vi "SS2 Live_Settings Storage.vi"(6 "Set/Get(F)":bool, 8 "Error In":errorcluster, 10 "Variant Data in":variant, 11 "Settings List":T8) -> (0 "Error Out":errorcluster, 2 "Variant Data out":variant)   [LabVIEW 2019]
uses:
  SS2 Live_Settings List.ctl
  SS2 DAQ Parameters 2.ctl
  SS2 Gate Definition.ctl
  SS2 Live_File Information.ctl
  SS2 Gate Configuration.ctl
  SS2 Live_Image ROI Information.ctl
  Phasor/Image Binning Options.ctl
  281105eb-bd69-41f7-a288-d5f8cce70846.vi
panel:
  in  "Tab Control":T1(tab)
  in  "Bitfile Version":string
  in  "BitFile Path":path
  in  "Buffer Size (# Gates)":u32=1 min=1
  in  "SS2 DAQ Parameters":T2 {"Laser Period" min=0.0 max=4.294967295}
  in  "Gate Configuration Definitions":T4[](array[typedef])
  in  "Image Binning Options":T5={"Use Image Binning"=FALSE, "X Bin"=1, "Y Bin"=1} {"Y Bin" min=1; "X Bin" min=1}
  in  "Image ROI Information":T6
  in  "# Datasets in Series":i32=1 min=1
  in  "File Information":T7
  in  "# Histogram Bins":i32=1 min=1 step=1
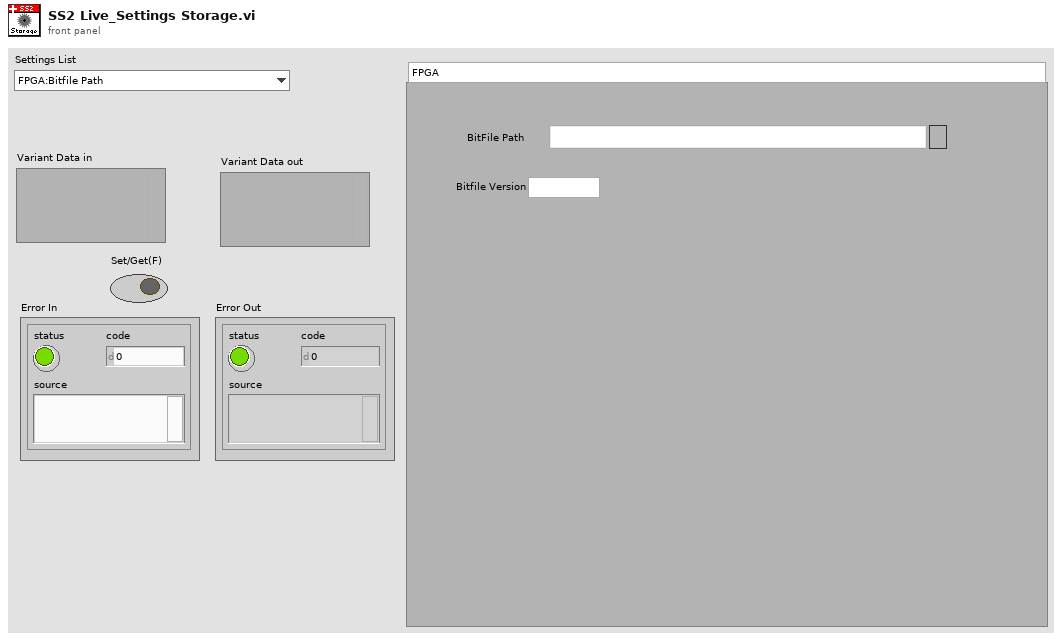
[diagram p1: front panel]
types:
  T1 = enum32{"FPGA", "Acquisition Parameters", "Image Parameters", "File Information", "UI Parameters"}
  T2 = typedef "SS2 DAQ Parameters 2.ctl" = cluster{"10 bits":bool, "# Exposure Sequences":u32, "# 1-bit Frame per Gate":u32, "Gate Shift":u32, "# Gates per Set":u32, "# Sets":u32, "Laser Period":dbl[unit], "Gate Offset":u32, "Auto-adjust Gate Offset":bool, "Gate Definition":T3}
  T3 = typedef "SS2 Gate Definition.ctl" = cluster{"gs_psincdec_0":u32, "gs_psincdec_1":u32, "gs_psincdec_2":u32, "gs_psincdec_3":u32, "gs_no_shift_adj_1":u32, "gs_no_shift_adj_2":u32, "gs_no_shift_adj_3":u32}
  T4 = typedef "SS2 Gate Configuration.ctl" = cluster{"Gate Configuration":string, "Gate Offset":u32, "Gate Definition":T3}
  T5 = typedef "Image Binning Options.ctl" = cluster{"Use Image Binning":bool, "X Bin":i32, "Y Bin":i32}
  T6 = typedef "SS2 Live_Image ROI Information.ctl" = cluster{"Save ROI Only":bool, "Left":u16, "Top":u16, "Right":u16, "Bottom":u16, "Use Current ROI":bool}
  T7 = typedef "SS2 Live_File Information.ctl" = cluster{"File Folder":path, "File Name":string, "File Index":u32, "Author":string, "Sample":string, "Compression":bool}
  T8 = typedef "SS2 Live_Settings List.ctl" = enum16{"FPGA:Bitfile Path", "FPGA:Bitfile Version", "Acquisition Parameters:SS2 DAQ Parameters", "Acquisition Parameters:Gate Configuration Array", "Acquisition Parameters:Buffer Size (# Gates)", "File Information:File Information", "File Information:# Datasets in Series", "Image Parameters:Image ROI Information", "Image Parameters:Image Binning Options", "UI Parameters:Histogram Bins Number"}
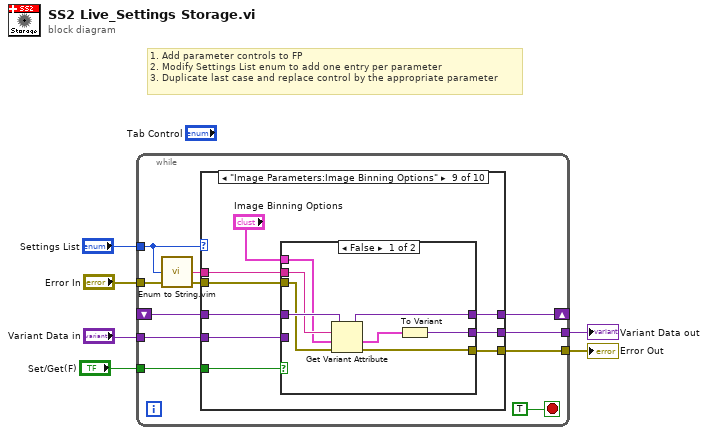
[diagram p0: block diagram]
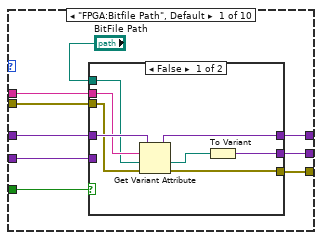
[diagram p2: hidden frame]
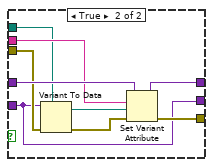
[diagram p3: hidden frame]
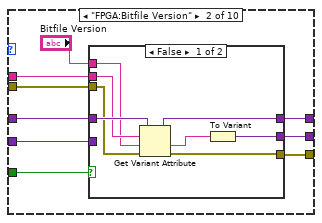
[diagram p4: hidden frame]
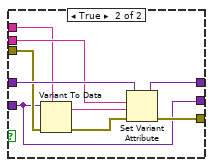
[diagram p5: hidden frame]
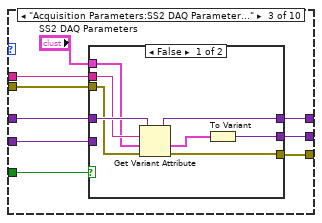
[diagram p6: hidden frame]
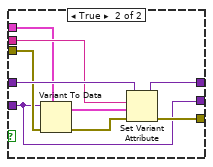
[diagram p7: hidden frame]
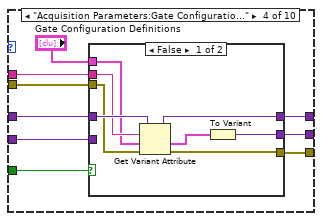
[diagram p8: hidden frame]
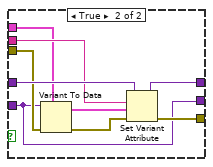
[diagram p9: hidden frame]
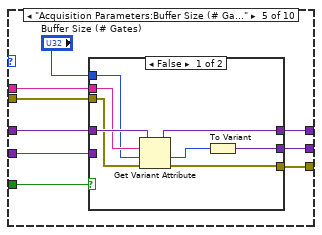
[diagram p10: hidden frame]
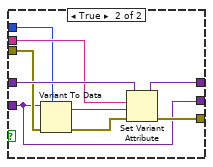
[diagram p11: hidden frame]
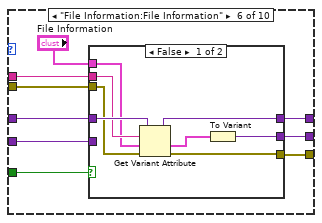
[diagram p12: hidden frame]
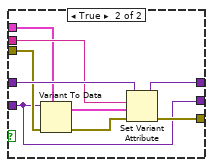
[diagram p13: hidden frame]
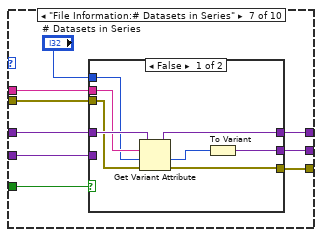
[diagram p14: hidden frame]
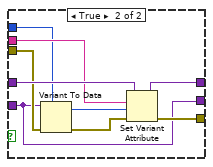
[diagram p15: hidden frame]
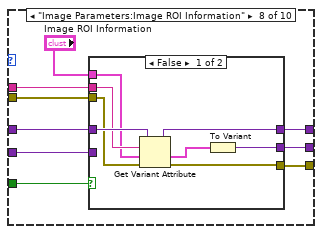
[diagram p16: hidden frame]
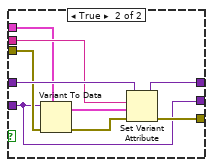
[diagram p17: hidden frame]
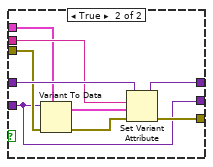
[diagram p18: hidden frame]
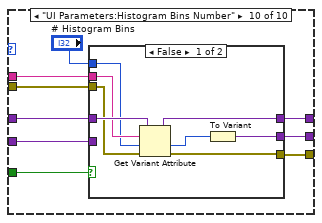
[diagram p19: hidden frame]
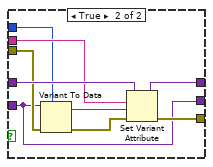
[diagram p20: hidden frame]
diagram:
  # "1. Add parameter controls to FP\n2. Modify Settings List enum to add one entry per parameter\n3. Duplicate last case and replace control by the appropriate parameter"
  n1 = while {
    tunnel: "Settings List" -> [w9]
    tunnel: "Error In" -> [w7]
    tunnel: "Set/Get(F)" -> [w15]
    shift-right: [w13] -> _
    shift-left: _ -> [w14]
    tunnel: "Variant Data in" -> [w12]
    tunnel: [w11] -> w2
    tunnel: [w10] -> w1
    stop <- TRUE stop-if-true
    n2 = call "Enum to String.vim"("Enum"=w9) -> ("String"=w8:string)
    n3 = case shown="\"Image Parameters:Image Binning Options\"" w9 {
      tunnel: w15 -> [w25 w51 w77 w103 w129 w155 w181 w207 w233 w259]
      tunnel: w14 -> [w24 w50 w76 w102 w128 w154 w180 w206 w232 w258]
      tunnel: w8 -> [w23 w49 w75 w101 w127 w153 w179 w205 w231 w257]
      tunnel: [w22 w48 w74 w100 w126 w152 w178 w204 w230 w256] -> w13
      tunnel: w7 -> [w21 w47 w73 w99 w125 w151 w177 w203 w229 w255]
      tunnel: w12 -> [w20 w46 w72 w98 w124 w150 w176 w202 w228 w254]
      tunnel: [w19 w45 w71 w97 w123 w149 w175 w201 w227 w253] -> w11
      tunnel: [w18 w44 w70 w96 w122 w148 w174 w200 w226 w252] -> w10
      frame "FPGA:Bitfile Path", Default {
        n4 = case shown="False" w25 {
          tunnel: w24 -> [w33 w42]
          tunnel: w23 -> [w32 w41]
          tunnel: [w30 w40] -> w22
          tunnel: "BitFile Path" -> [w27 w39]
          tunnel: w21 -> [w31 w38]
          tunnel: w20 -> [_ w34]
          tunnel: [w29 w35] -> w19
          tunnel: [w26 w34] -> w18
          frame False {
            n5 = Get Variant Attribute(Variant=w33, name=w32, default value (empty Variant)=w27, error in=w31) -> (duplicate Variant=w30:variant, value=w28:path, error out=w29:errorcluster)  [unwired: 1 out]
            n6 = To Variant(anything=w28) -> (Variant=w26:variant)
          }
          frame True {
            n7 = Variant To Data(error in=w38, type=w39, Variant=w34) -> (data=w37:path, error out=w36:errorcluster)
            n8 = Set Variant Attribute(Variant=w42, name=w41, value=w37, error in=w36) -> (Variant out=w40:variant, error out=w35:errorcluster)  [unwired: 1 out]
          }
        }
      }
      frame "FPGA:Bitfile Version" {
        n9 = case shown="False" w51 {
          tunnel: w50 -> [w59 w68]
          tunnel: w49 -> [w58 w67]
          tunnel: [w56 w66] -> w48
          tunnel: "Bitfile Version" -> [w53 w65]
          tunnel: w47 -> [w57 w64]
          tunnel: w46 -> [_ w60]
          tunnel: [w55 w61] -> w45
          tunnel: [w52 w60] -> w44
          frame False {
            n10 = Get Variant Attribute(Variant=w59, name=w58, default value (empty Variant)=w53, error in=w57) -> (duplicate Variant=w56:variant, value=w54:string, error out=w55:errorcluster)  [unwired: 1 out]
            n11 = To Variant(anything=w54) -> (Variant=w52:variant)
          }
          frame True {
            n12 = Variant To Data(error in=w64, type=w65, Variant=w60) -> (data=w63:string, error out=w62:errorcluster)
            n13 = Set Variant Attribute(Variant=w68, name=w67, value=w63, error in=w62) -> (Variant out=w66:variant, error out=w61:errorcluster)  [unwired: 1 out]
          }
        }
      }
      frame "Acquisition Parameters:SS2 DAQ Parameters" {
        n14 = case shown="False" w77 {
          tunnel: w76 -> [w85 w94]
          tunnel: w75 -> [w84 w93]
          tunnel: [w82 w92] -> w74
          tunnel: "SS2 DAQ Parameters" -> [w79 w91]
          tunnel: w73 -> [w83 w90]
          tunnel: w72 -> [_ w86]
          tunnel: [w81 w87] -> w71
          tunnel: [w78 w86] -> w70
          frame False {
            n15 = Get Variant Attribute(Variant=w85, name=w84, default value (empty Variant)=w79, error in=w83) -> (duplicate Variant=w82:variant, value=w80:T2, error out=w81:errorcluster)  [unwired: 1 out]
            n16 = To Variant(anything=w80) -> (Variant=w78:variant)
          }
          frame True {
            n17 = Variant To Data(error in=w90, type=w91, Variant=w86) -> (data=w89:T2, error out=w88:errorcluster)
            n18 = Set Variant Attribute(Variant=w94, name=w93, value=w89, error in=w88) -> (Variant out=w92:variant, error out=w87:errorcluster)  [unwired: 1 out]
          }
        }
      }
      frame "Acquisition Parameters:Gate Configuration Array" {
        n19 = case shown="False" w103 {
          tunnel: w102 -> [w111 w120]
          tunnel: w101 -> [w110 w119]
          tunnel: [w108 w118] -> w100
          tunnel: "Gate Configuration Definitions" -> [w105 w117]
          tunnel: w99 -> [w109 w116]
          tunnel: w98 -> [_ w112]
          tunnel: [w107 w113] -> w97
          tunnel: [w104 w112] -> w96
          frame False {
            n20 = Get Variant Attribute(Variant=w111, name=w110, default value (empty Variant)=w105, error in=w109) -> (duplicate Variant=w108:variant, value=w106:T4[], error out=w107:errorcluster)  [unwired: 1 out]
            n21 = To Variant(anything=w106) -> (Variant=w104:variant)
          }
          frame True {
            n22 = Variant To Data(error in=w116, type=w117, Variant=w112) -> (data=w115:T4[], error out=w114:errorcluster)
            n23 = Set Variant Attribute(Variant=w120, name=w119, value=w115, error in=w114) -> (Variant out=w118:variant, error out=w113:errorcluster)  [unwired: 1 out]
          }
        }
      }
      frame "Acquisition Parameters:Buffer Size (# Gates)" {
        n24 = case shown="False" w129 {
          tunnel: w128 -> [w137 w146]
          tunnel: w127 -> [w136 w145]
          tunnel: [w134 w144] -> w126
          tunnel: "Buffer Size (# Gates)" -> [w131 w143]
          tunnel: w125 -> [w135 w142]
          tunnel: w124 -> [_ w138]
          tunnel: [w133 w139] -> w123
          tunnel: [w130 w138] -> w122
          frame False {
            n25 = Get Variant Attribute(Variant=w137, name=w136, default value (empty Variant)=w131, error in=w135) -> (duplicate Variant=w134:variant, value=w132:u32, error out=w133:errorcluster)  [unwired: 1 out]
            n26 = To Variant(anything=w132) -> (Variant=w130:variant)
          }
          frame True {
            n27 = Variant To Data(error in=w142, type=w143, Variant=w138) -> (data=w141:u32, error out=w140:errorcluster)
            n28 = Set Variant Attribute(Variant=w146, name=w145, value=w141, error in=w140) -> (Variant out=w144:variant, error out=w139:errorcluster)  [unwired: 1 out]
          }
        }
      }
      frame "File Information:File Information" {
        n29 = case shown="False" w155 {
          tunnel: w154 -> [w163 w172]
          tunnel: w153 -> [w162 w171]
          tunnel: [w160 w170] -> w152
          tunnel: "File Information" -> [w157 w169]
          tunnel: w151 -> [w161 w168]
          tunnel: w150 -> [_ w164]
          tunnel: [w159 w165] -> w149
          tunnel: [w156 w164] -> w148
          frame False {
            n30 = Get Variant Attribute(Variant=w163, name=w162, default value (empty Variant)=w157, error in=w161) -> (duplicate Variant=w160:variant, value=w158:T7, error out=w159:errorcluster)  [unwired: 1 out]
            n31 = To Variant(anything=w158) -> (Variant=w156:variant)
          }
          frame True {
            n32 = Variant To Data(error in=w168, type=w169, Variant=w164) -> (data=w167:T7, error out=w166:errorcluster)
            n33 = Set Variant Attribute(Variant=w172, name=w171, value=w167, error in=w166) -> (Variant out=w170:variant, error out=w165:errorcluster)  [unwired: 1 out]
          }
        }
      }
      frame "File Information:# Datasets in Series" {
        n34 = case shown="False" w181 {
          tunnel: w180 -> [w189 w198]
          tunnel: w179 -> [w188 w197]
          tunnel: [w186 w196] -> w178
          tunnel: "# Datasets in Series" -> [w183 w195]
          tunnel: w177 -> [w187 w194]
          tunnel: w176 -> [_ w190]
          tunnel: [w185 w191] -> w175
          tunnel: [w182 w190] -> w174
          frame False {
            n35 = Get Variant Attribute(Variant=w189, name=w188, default value (empty Variant)=w183, error in=w187) -> (duplicate Variant=w186:variant, value=w184:i32, error out=w185:errorcluster)  [unwired: 1 out]
            n36 = To Variant(anything=w184) -> (Variant=w182:variant)
          }
          frame True {
            n37 = Variant To Data(error in=w194, type=w195, Variant=w190) -> (data=w193:i32, error out=w192:errorcluster)
            n38 = Set Variant Attribute(Variant=w198, name=w197, value=w193, error in=w192) -> (Variant out=w196:variant, error out=w191:errorcluster)  [unwired: 1 out]
          }
        }
      }
      frame "Image Parameters:Image ROI Information" {
        n39 = case shown="False" w207 {
          tunnel: w206 -> [w215 w224]
          tunnel: w205 -> [w214 w223]
          tunnel: [w212 w222] -> w204
          tunnel: "Image ROI Information" -> [w209 w221]
          tunnel: w203 -> [w213 w220]
          tunnel: w202 -> [_ w216]
          tunnel: [w211 w217] -> w201
          tunnel: [w208 w216] -> w200
          frame False {
            n40 = Get Variant Attribute(Variant=w215, name=w214, default value (empty Variant)=w209, error in=w213) -> (duplicate Variant=w212:variant, value=w210:T6, error out=w211:errorcluster)  [unwired: 1 out]
            n41 = To Variant(anything=w210) -> (Variant=w208:variant)
          }
          frame True {
            n42 = Variant To Data(error in=w220, type=w221, Variant=w216) -> (data=w219:T6, error out=w218:errorcluster)
            n43 = Set Variant Attribute(Variant=w224, name=w223, value=w219, error in=w218) -> (Variant out=w222:variant, error out=w217:errorcluster)  [unwired: 1 out]
          }
        }
      }
      frame "Image Parameters:Image Binning Options" {
        n44 = case shown="False" w233 {
          tunnel: w232 -> [w241 w250]
          tunnel: w231 -> [w240 w249]
          tunnel: [w238 w248] -> w230
          tunnel: "Image Binning Options" -> [w235 w247]
          tunnel: w229 -> [w239 w246]
          tunnel: w228 -> [_ w242]
          tunnel: [w237 w243] -> w227
          tunnel: [w234 w242] -> w226
          frame False {
            n45 = Get Variant Attribute(Variant=w241, name=w240, default value (empty Variant)=w235, error in=w239) -> (duplicate Variant=w238:variant, value=w236:T5, error out=w237:errorcluster)  [unwired: 1 out]
            n46 = To Variant(anything=w236) -> (Variant=w234:variant)
          }
          frame True {
            n47 = Variant To Data(error in=w246, type=w247, Variant=w242) -> (data=w245:T5, error out=w244:errorcluster)
            n48 = Set Variant Attribute(Variant=w250, name=w249, value=w245, error in=w244) -> (Variant out=w248:variant, error out=w243:errorcluster)  [unwired: 1 out]
          }
        }
      }
      frame "UI Parameters:Histogram Bins Number" {
        n49 = case shown="False" w259 {
          tunnel: w258 -> [w267 w276]
          tunnel: w257 -> [w266 w275]
          tunnel: [w264 w274] -> w256
          tunnel: "# Histogram Bins" -> [w261 w273]
          tunnel: w255 -> [w265 w272]
          tunnel: w254 -> [_ w268]
          tunnel: [w263 w269] -> w253
          tunnel: [w260 w268] -> w252
          frame False {
            n50 = Get Variant Attribute(Variant=w267, name=w266, default value (empty Variant)=w261, error in=w265) -> (duplicate Variant=w264:variant, value=w262:i32, error out=w263:errorcluster)  [unwired: 1 out]
            n51 = To Variant(anything=w262) -> (Variant=w260:variant)
          }
          frame True {
            n52 = Variant To Data(error in=w272, type=w273, Variant=w268) -> (data=w271:i32, error out=w270:errorcluster)
            n53 = Set Variant Attribute(Variant=w276, name=w275, value=w271, error in=w270) -> (Variant out=w274:variant, error out=w269:errorcluster)  [unwired: 1 out]
          }
        }
      }
    }
  }
  "Error Out" <- w2
  "Variant Data out" <- w1
